vi "Flipping_Four_Coins.vi"() -> ()   [LabVIEW 2022 SP3]
uses:
  <vilib>/Analysis/NI_AALBase.lvlib
panel:
  out "XY Graph":T1(graph)
  in  "Total Number of Trials":i32
  out "Number of Heads":dbl
  out "Coin 4":bool
  out "Coin 3":bool
  out "Coin 2":bool
  out "Coin 1":bool
  # "Flipping_Four_Coins:\nEnter a number into the \"Total Number of Trials\" box\nfor 4 coins to be flipped that many times. The number \nof heads for each trial will be displayed below, and a bar chart\nwill be populated showing the number of trials that resulted in\n0, 1, 2, 3, and 4 heads."
  # "Heads = Lit"
  # "Tails = Unlit"
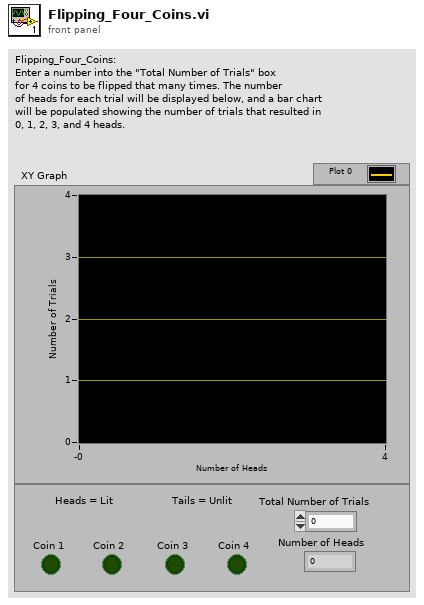
[diagram p1: front panel]
types:
  T1 = cluster{"X Values":dbl[], "Histogram: h(x)":i32[]}
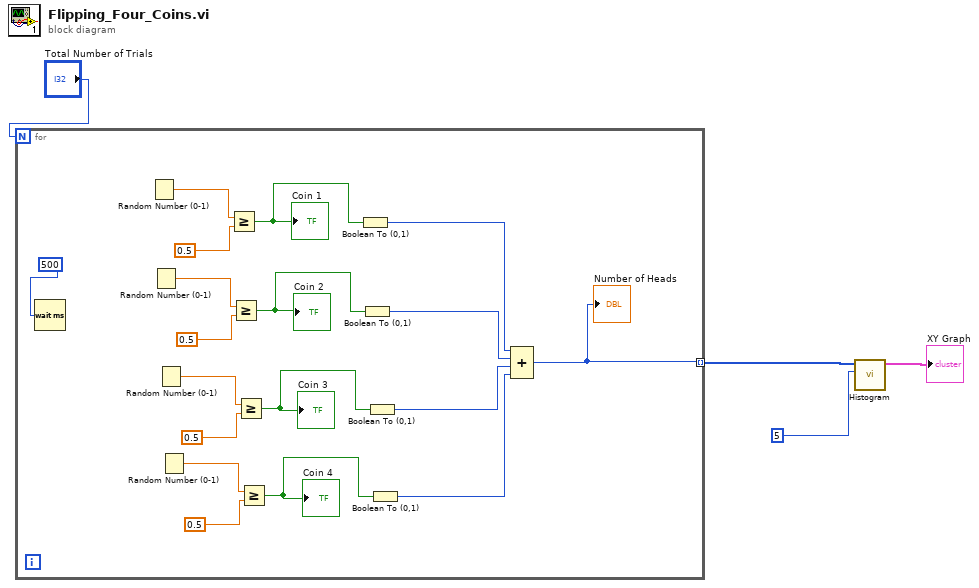
[diagram p0: block diagram]
diagram:
  n1 = for {
    N: "Total Number of Trials" -> [_]
    tunnel: [w5] -> w3 mode=indexing
    n2 = Wait (ms)(milliseconds to wait=500) -> ()  [unwired: 1 out]
    n3 = Random Number (0-1)() -> (number: 0 to 1=w22:dbl)
    n4 = Random Number (0-1)() -> (number: 0 to 1=w16:dbl)
    n5 = Random Number (0-1)() -> (number: 0 to 1=w20:dbl)
    n6 = Random Number (0-1)() -> (number: 0 to 1=w18:dbl)
    n7 = Greater Or Equal?(x=w22, y=0.5) -> (x >= y?=w11:bool)
    "Coin 1" <- w11
    n8 = Greater Or Equal?(x=w16, y=0.5) -> (x >= y?=w12:bool)
    "Coin 2" <- w12
    n9 = Greater Or Equal?(x=w20, y=0.5) -> (x >= y?=w13:bool)
    "Coin 3" <- w13
    n10 = Greater Or Equal?(x=w18, y=0.5) -> (x >= y?=w14:bool)
    "Coin 4" <- w14
    n11 = Boolean To (0,1)(Boolean=w11) -> (0, 1=w10:i16)
    n12 = Boolean To (0,1)(Boolean=w12) -> (0, 1=w8:i16)
    n13 = Boolean To (0,1)(Boolean=w13) -> (0, 1=w7:i16)
    n14 = Boolean To (0,1)(Boolean=w14) -> (0, 1=w9:i16)
    n15 = Compound Arithmetic op=ADD(w10, w8, w7, w9) -> (w5:i16)
    "Number of Heads" <- w5
  }
  n16 = call <vilib>:"Histogram.vi"("intervals"=5, "X"=w3) -> ("Histogram Graph"=→"XY Graph":T1)  [unwired: 6 in, 3 out]
